vi "GetLabelText.vi"(0 "reference in":refnum<class "Control.lvclass">, 5 "error in (no error)":errorcluster) -> (14 "reference out":refnum<class "Control.lvclass">, 16 "Text":string, 19 "error out":errorcluster)   [LabVIEW 2014, in "FrontPanelPublisher.lvlib" / "Control.lvclass"]
uses:
  Control.lvclass
  Text_class/Text.lvclass
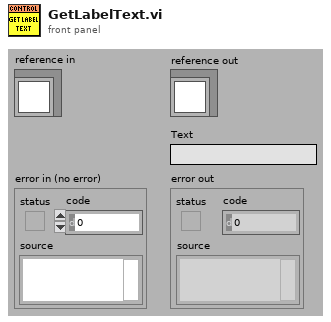
[diagram p1: front panel]
types:
  T1 = typedef "FrontPanelPublisher.lvlib/Control.lvclass/Attributes.ctl" = cluster{"Description":string, "Indicator":bool, "Default Value":variant, "Control Index":i32, "Label":refnum<class "Text.lvclass">, "Caption":refnum<class "Text.lvclass">, "Use Picture":bool, "Image1 b64":string, "Image2 b64":string}
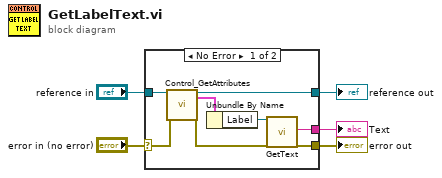
[diagram p0: block diagram]
diagram:
  n1 = case shown="No Error" "error in (no error)" {
    selector: "error in (no error)" -> [w13 w15]
    tunnel: [w7 w15] -> w4
    tunnel: [w10 w14] -> w2
    tunnel: "reference in" -> [w11 w14]
    tunnel: [w6 _] -> w1
    frame No Error {
      n2 = call "Control_GetAttributes.vi"("reference in"=w11, "error in (no error)"=w13) -> ("reference out"=w10:refnum<class "Control.lvclass">, "Data"=w12:T1, "error out"=w8:errorcluster)  [unwired: 14 in, 1 out]
      n3 = Unbundle By Name(w12) -> ("Label"=w9:refnum<class "Text.lvclass">)
      n4 = call-dynamic "GetText.vi"("reference in"=w9, "error in (no error)"=w8) -> ("Text"=w6:string, "error out"=w7:errorcluster)  [unwired: 15 in, 1 out]
    }
    frame Error {
    }
  }
  "error out" <- w4
  "reference out" <- w2
  "Text" <- w1
